vi "ForceGraph.vi"(6 "Boolean":bool, 8 "number":dbl, 9 "Setpoint":dbl, 10 "k":dbl, 11 "Function":string) -> (1 "force":dbl)   [LabVIEW 2022 SP3]
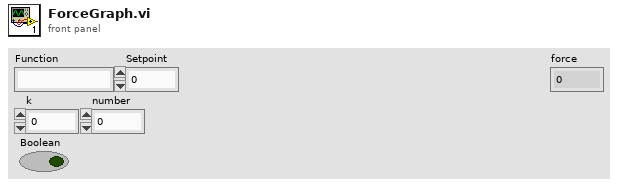
[diagram p1: front panel]
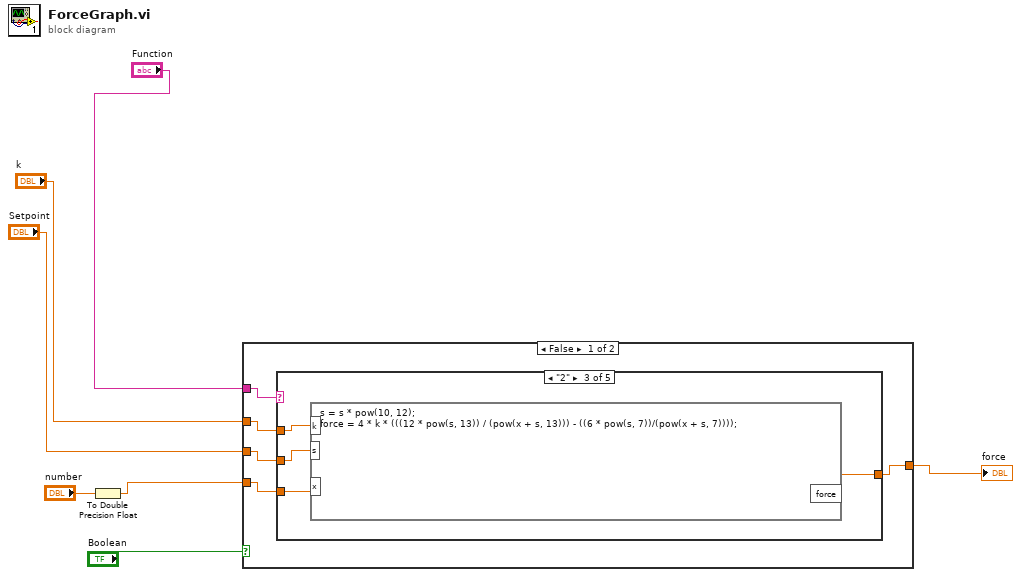
[diagram p0: block diagram]
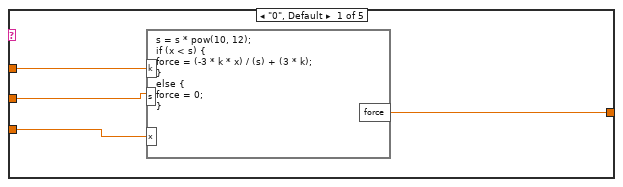
[diagram p2: hidden frame]
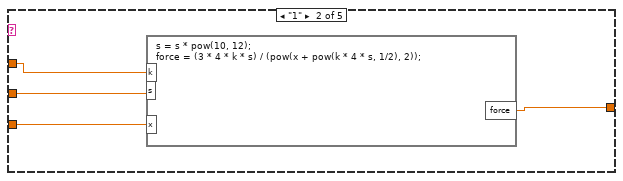
[diagram p3: hidden frame]
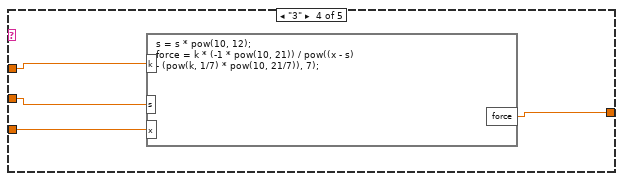
[diagram p4: hidden frame]
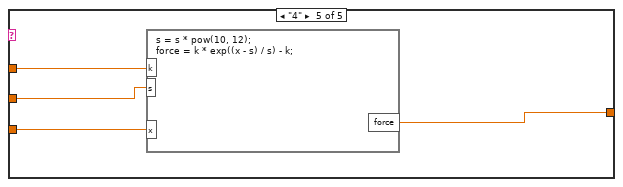
[diagram p5: hidden frame]
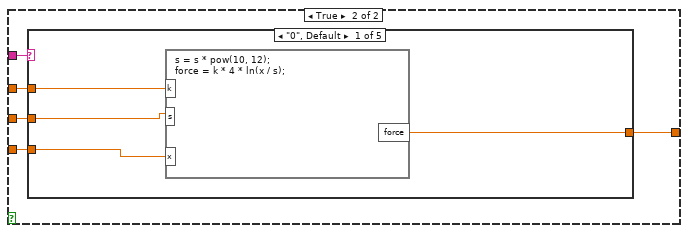
[diagram p6: hidden frame]
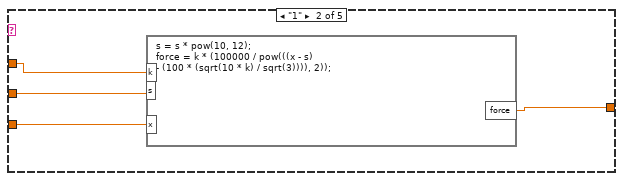
[diagram p7: hidden frame]
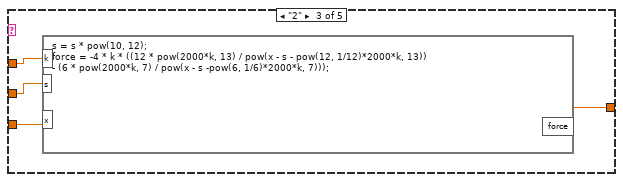
[diagram p8: hidden frame]
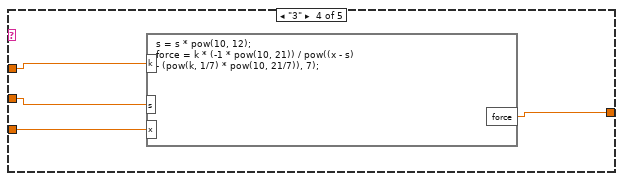
[diagram p9: hidden frame]
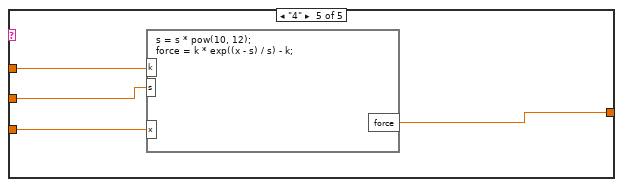
[diagram p10: hidden frame]
diagram:
  n1 = To Double Precision Float(number="number") -> (double precision float=w4:dbl)
  n2 = case shown="False" "Boolean" {
    tunnel: "Function" -> [w10 w37]
    tunnel: "Setpoint" -> [w9 w36]
    tunnel: "k" -> [w11 w35]
    tunnel: w4 -> [w8 w34]
    tunnel: [w12 w33] -> w2
    frame False {
      n3 = case shown="\"2\"" w10 {
        tunnel: [w15 w19 w23 w28 w31] -> w12
        tunnel: w8 -> [w16 w20 w24 w27 w32]
        tunnel: w9 -> [w14 w17 w21 w25 w29]
        tunnel: w11 -> [w13 w18 w22 w26 w30]
        frame "0", Default {
          n4 = formula code="s = s * pow(10, 12);\nif (x < s) {\nforce = (-3 * k * x) / (s) + (3 * k);\n}\nelse {\nforce = 0;\n}"("k"=w13, "s"=w14, "x"=w16) -> ("force"=w15:dbl)
        }
        frame "1" {
          n5 = formula code="s = s * pow(10, 12);\nforce = (3 * 4 * k * s) / (pow(x + pow(k * 4 * s, 1/2), 2));"("k"=w18, "s"=w17, "x"=w20) -> ("force"=w19:dbl)
        }
        frame "2" {
          n6 = formula code="s = s * pow(10, 12);\nforce = 4 * k * (((12 * pow(s, 13)) / (pow(x + s, 13))) - ((6 * pow(s, 7))/(pow(x + s, 7))));"("x"=w24, "s"=w21, "k"=w22) -> ("force"=w23:dbl)
        }
        frame "3" {
          n7 = formula code="s = s * pow(10, 12);\nforce = k * (-1 * pow(10, 21)) / pow((x - s) \n- (pow(k, 1/7) * pow(10, 21/7)), 7);"("k"=w26, "s"=w25, "x"=w27) -> ("force"=w28:dbl)
        }
        frame "4" {
          n8 = formula code="s = s * pow(10, 12);\nforce = k * exp((x - s) / s) - k;"("k"=w30, "s"=w29, "x"=w32) -> ("force"=w31:dbl)
        }
      }
    }
    frame True {
      n9 = case shown="\"0\", Default" w37 {
        tunnel: [w40 w44 w48 w53 w56] -> w33
        tunnel: w34 -> [w41 w45 w49 w52 w57]
        tunnel: w36 -> [w39 w42 w46 w50 w54]
        tunnel: w35 -> [w38 w43 w47 w51 w55]
        frame "0", Default {
          n10 = formula code="s = s * pow(10, 12);\nforce = k * 4 * ln(x / s);"("k"=w38, "s"=w39, "x"=w41) -> ("force"=w40:dbl)
        }
        frame "1" {
          n11 = formula code="s = s * pow(10, 12);\nforce = k * (100000 / pow(((x - s) \n- (100 * (sqrt(10 * k) / sqrt(3)))), 2));"("k"=w43, "s"=w42, "x"=w45) -> ("force"=w44:dbl)
        }
        frame "2" {
          n12 = formula code="s = s * pow(10, 12);\nforce = -4 * k * ((12 * pow(2000*k, 13) / pow(x - s - pow(12, 1/12)*2000*k, 13)) \n- (6 * pow(2000*k, 7) / pow(x - s -pow(6, 1/6)*2000*k, 7)));"("x"=w49, "s"=w46, "k"=w47) -> ("force"=w48:dbl)
        }
        frame "3" {
          n13 = formula code="s = s * pow(10, 12);\nforce = k * (-1 * pow(10, 21)) / pow((x - s) \n- (pow(k, 1/7) * pow(10, 21/7)), 7);"("k"=w51, "s"=w50, "x"=w52) -> ("force"=w53:dbl)
        }
        frame "4" {
          n14 = formula code="s = s * pow(10, 12);\nforce = k * exp((x - s) / s) - k;"("k"=w55, "s"=w54, "x"=w57) -> ("force"=w56:dbl)
        }
      }
    }
  }
  "force" <- w2
